vi "Gas Flow Readings.vi"(0 "Com Flow Computer":refnum<visa-resource-name>, 1 "task/channels in":refnum<k21>="PortRead", 5 "Use SL9200 Gas Readings?":bool, 7 "Use Dry Gas Meter?":bool=TRUE, 9 "Initialize?":bool=TRUE, 11 "Error In":errorcluster, 12 "Encoder":T1={"ft3 Per Rotation"=0.1, "Ticks Per Rotation"=400.0, "Data Sample Period(mS)"=10, "Number of Samples"=50} {"ft3 Per Rotation" format="%_3g"}) -> (4 "Labels":string[](array[string]), 6 "Values":string[](array[string]), 15 "error out":errorcluster)   [LabVIEW 2012]
uses:
  SL9200 Flow Calc/SL9200_Registers.ctl
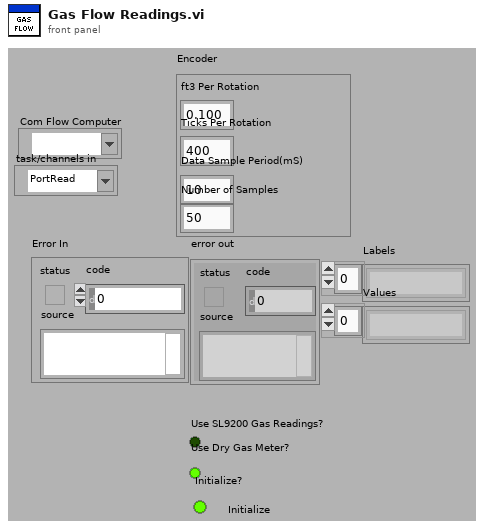
[diagram p1: front panel]
types:
  T1 = cluster{"ft3 Per Rotation":dbl, "Ticks Per Rotation":dbl, "Data Sample Period(mS)":u32, "Number of Samples":i32}
  T2 = typedef "SL9200_Registers.ctl" = u8
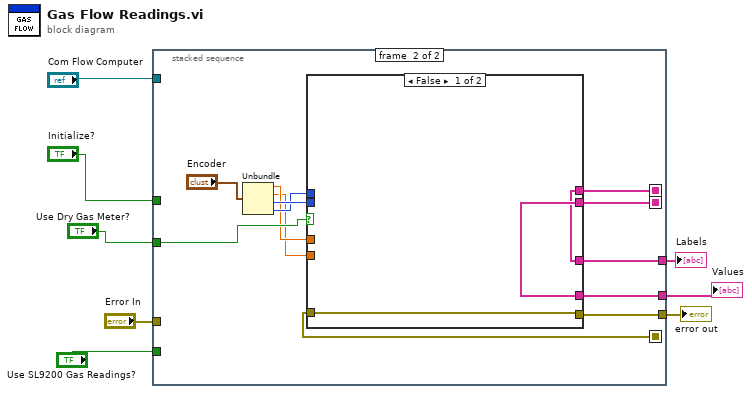
[diagram p0: block diagram]
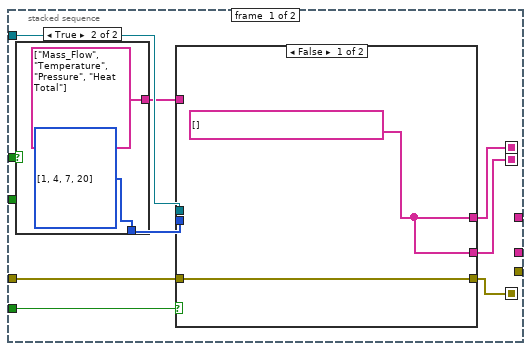
[diagram p2: hidden frame]
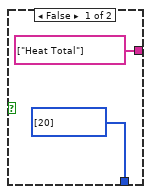
[diagram p3: hidden frame]
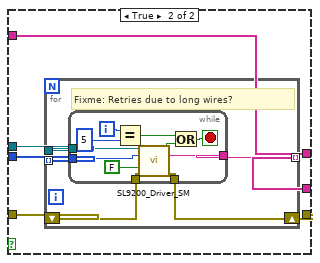
[diagram p4: hidden frame]
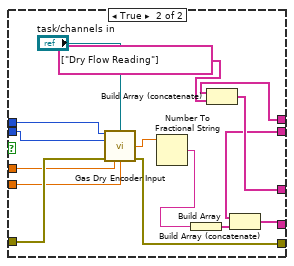
[diagram p5: hidden frame]
diagram:
  n1 = stacked-sequence {
    seq-local: [w15 _] -> [_ w57]
    seq-local: [w14 _] -> [_ w55]
    seq-local: [w12 _] -> [_ w52]
    tunnel: "Error In" -> [w16 _]
    tunnel: [_ w54] -> w2
    tunnel: [_ w56] -> w3
    tunnel: "Use SL9200 Gas Readings?" -> [w13 _]
    tunnel: "Use Dry Gas Meter?" -> [_ w53]
    tunnel: [_ w51] -> w5
    tunnel: "Com Flow Computer" -> [w11 _]
    tunnel: "Initialize?" -> [w10 _]
    frame #0 {
      n2 = case shown="True" w10 {
        tunnel: [w19 w21] -> w17
        tunnel: [string[] ["Heat Total"] ("array") string[] ["Mass_Flow", "Temperature", "Pressure", "Heat Total"] ("array")] -> w9
        frame False {
          w19 = T2[] [20] items=["Heat_Flow", "Mass_Flow", "Corrected_Volume_Flow", "Volume_Flow", "Temperature", "Temperature2", "Delta_Temperature", "Pressure", "Diff_Pressure", "Density", "Spec_Enthalpy", "Date", "Time", "Level", "Peak_Demand", "Demand_Last_Hour", "Peak_Demand_Time", "Peak_Demand_Date", "Viscosity", "Reynolds_Number", "Heat_Total", "Grand_Heat_Total", "Mass_Total", "Grand_Mass", "Corrected_Volume_Total", "Grand_Corrected_Volume", "Volume_Total", "Grand_Volume", "Totalizer_Reset", "Alarm_Reset", "Barometric", "Fluid_Type", "Reference_Density", "Therm_Expansion_Coef", "Combustion_Heat", "Specific_Heat", "Flow_Z_Factor", "Ref_Z_Factor", "Isentropic_Exponent", "Viscosity_A", "Viscosity_B", "Reference_Temperature", "Calibration_Density", "Base_Density_H2O_4C", "Per_Mole_N2", "Per_Mole_CO2", "Tag_Number", "Software_Version", "Hardware_Version", "Order_Code", "Serial_Number", "Sensor_Serial_Num"]
        }
        frame True {
          w21 = T2[] [1, 4, 7, 20] items=["Heat_Flow", "Mass_Flow", "Corrected_Volume_Flow", "Volume_Flow", "Temperature", "Temperature2", "Delta_Temperature", "Pressure", "Diff_Pressure", "Density", "Spec_Enthalpy", "Date", "Time", "Level", "Peak_Demand", "Demand_Last_Hour", "Peak_Demand_Time", "Peak_Demand_Date", "Viscosity", "Reynolds_Number", "Heat_Total", "Grand_Heat_Total", "Mass_Total", "Grand_Mass", "Corrected_Volume_Total", "Grand_Corrected_Volume", "Volume_Total", "Grand_Volume", "Totalizer_Reset", "Alarm_Reset", "Barometric", "Fluid_Type", "Reference_Density", "Therm_Expansion_Coef", "Combustion_Heat", "Specific_Heat", "Flow_Z_Factor", "Ref_Z_Factor", "Isentropic_Exponent", "Viscosity_A", "Viscosity_B", "Reference_Temperature", "Calibration_Density", "Base_Density_H2O_4C", "Per_Mole_N2", "Per_Mole_CO2", "Tag_Number", "Software_Version", "Hardware_Version", "Order_Code", "Serial_Number", "Sensor_Serial_Num"]
        }
      }
      n3 = case shown="False" w13 {
        tunnel: w17 -> [_ w29]
        tunnel: w16 -> [w23 w28]
        tunnel: w11 -> [_ w27]
        tunnel: [w23 w26] -> w12
        tunnel: [w22 w25] -> w14
        tunnel: [w22 w24] -> w15
        tunnel: w9 -> [_ w24]
        frame False {
          w22 = string[] [] ("array")
        }
        frame True {
          n4 = for {
            tunnel: w27 -> [w34]
            tunnel: [w33] -> w25 mode=indexing
            tunnel: w29 -> [w32] mode=indexing
            shift-right: [w30] -> w26
            shift-left: w28 -> [w31]
            # "Fixme: Retries due to long wires?"
            n5 = while {
              tunnel: w34 -> [w45]
              tunnel: [w44] -> w33
              tunnel: w32 -> [w43]
              tunnel: w31 -> [w42]
              tunnel: [w41] -> w30
              i -> [w38]
              stop <- w35 stop-if-true
              n6 = Equal?(x=w38, y=5) -> (x = y?=w36:bool)
              n7 = call "SL9200_Driver_SM.vi"("ComPort"=w45, "Register"=w43, "InitSerial?"=FALSE, "Error In"=w42) -> ("CMD OK"=w39:bool, "Response"=w44:string, "Error Out"=w41:errorcluster)  [unwired: 9 in]
              n8 = Or(x=w36, y=w39) -> (x .or. y?=w35:bool)
            }
          }
        }
      }
    }
    frame #1 {
      n9 = Unbundle("Encoder") -> ("ft3 Per Rotation"=w47:dbl, "Ticks Per Rotation"=w46:dbl, "Data Sample Period(mS)"=w49:u32, "Number of Samples"=w48:i32)
      n10 = case shown="False" w53 {
        tunnel: w52 -> [w60 w75]
        tunnel: w57 -> [w58 w74]
        tunnel: [w58 w71] -> w56
        tunnel: w55 -> [w59 w70]
        tunnel: [w59 w69] -> w54
        tunnel: [w60 w66] -> w51
        tunnel: w49 -> [_ w64]
        tunnel: w48 -> [_ w63]
        tunnel: w47 -> [_ w62]
        tunnel: w46 -> [_ w61]
        frame False {
        }
        frame True {
          n11 = call "Gas Dry Encoder Input.vi"("Number of Samples"=w63, "task/channels in"="task/channels in", "Data Sample Period(mS)"=w64, "error in (no error)"=w75, "ft3 Per Rotation"=w62, "Ticks Per Rotation"=w61) -> ("ft3 per Hour"=w72:dbl, "error out"=w66:errorcluster)  [unwired: 6 in, 2 out]
          n12 = Number To Fractional String(number=w72) -> (F-format string=w67:string)  [unwired: 3 in]
          n13 = Build Array(w67) -> (w68:string[])
          n14 = Build Array (concatenate)(w74, string[] ["Dry Flow Reading"] ("array")) -> (w71:string[])
          n15 = Build Array (concatenate)(w70, w68) -> (w69:string[])
        }
      }
    }
  }
  "error out" <- w5
  "Labels" <- w3
  "Values" <- w2
